vi "Pre-Build Action.vi"(6 "Top Level/Always Included VIs":path[](array[path]), 7 "Main Destination Path":path, 9 "Target Name":string, 10 "Build Specification Name":string, 11 "Project Path":path) -> (0 "error out":errorcluster)   [LabVIEW 2023]
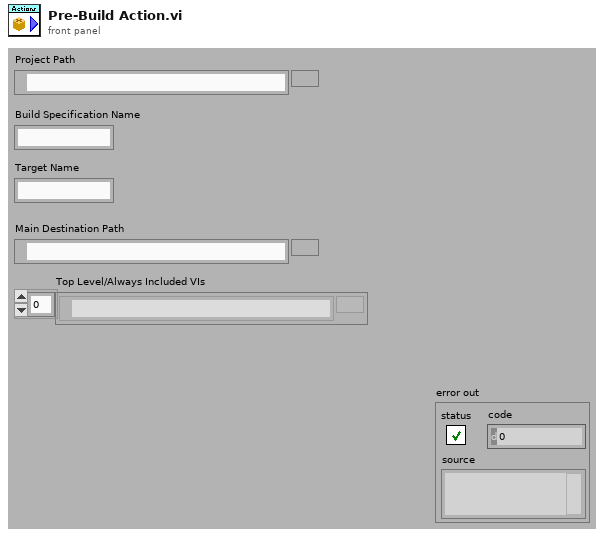
[diagram p1: front panel]
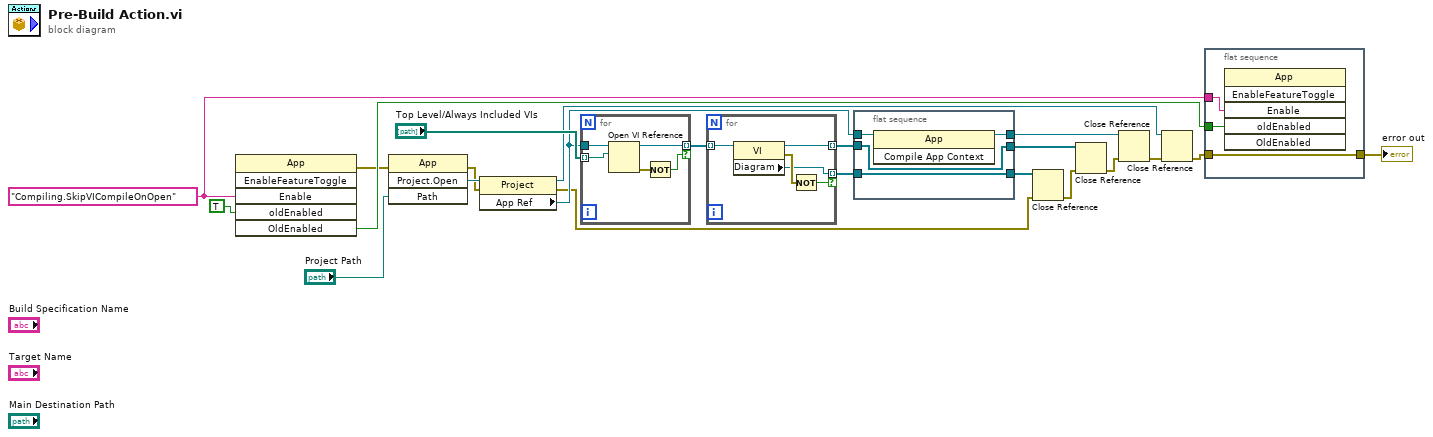
[diagram p0: block diagram]
diagram:
  w18 = "Compiling.SkipVICompileOnOpen" ("TokenName")
  n1 = invoke class="App" method="EnableFeatureToggle"("Enable"=w18, "oldEnabled"=TRUE ("Enable")) -> (error out=w16:errorcluster, "OldEnabled"=w17:bool)  [unwired: 4 in, 4 out]
  n2 = invoke class="App" method="Project.Open"(error in=w16, "Path"="Project Path") -> (error out=w20:errorcluster, "Project:Open"=w21:refnum<vi>)  [unwired: 2 in, 2 out]
  n3 = property class="Project"(reference=w21, error in=w20) -> (reference out=w5:refnum<vi>, error out=w4:errorcluster, "App Ref"=w11:refnum<vi>)
  n4 = for {
    tunnel: "Top Level/Always Included VIs" -> [w27] mode=indexing
    tunnel: [w26] -> w14 mode=indexing if=w24
    tunnel: w11 -> [w23]
    n5 = Open VI Reference(application reference (local)=w23, vi path=w27) -> (vi reference=w26:refnum<vi>, error out=w25:errorcluster)  [unwired: 4 in]
    n6 = Not(x=w25) -> (.not. x?=w24:bool)
  }
  n7 = for {
    tunnel: w14 -> [w32] mode=indexing
    tunnel: [w30] -> w12 mode=indexing if=w28
    tunnel: [w29] -> w13 mode=indexing
    n8 = property class="VI"(reference=w32) -> (reference out=w29:refnum<vi>, error out=w31:errorcluster, "Diagram"=w30:refnum<vi>)  [unwired: 1 in]
    n9 = Not(x=w31) -> (.not. x?=w28:bool)
  }
  n10 = flat-sequence {
    tunnel: [w36] -> w8
    tunnel: w13 -> [w36]
    tunnel: [w35] -> w10
    tunnel: w12 -> [w35]
    tunnel: w11 -> [w34]
    tunnel: [w33] -> w1
    frame #0 {
      n11 = invoke class="App" method="Compile App Context"(reference=w34) -> (reference out=w33:refnum<vi>)  [unwired: 2 in, 2 out]
    }
  }
  n12 = Close Reference(reference=w10, error in (no error)=w4) -> (error out=w9:errorcluster)
  n13 = Close Reference(reference=w8, error in (no error)=w9) -> (error out=w3:errorcluster)
  n14 = Close Reference(reference=w1, error in (no error)=w3) -> (error out=w2:errorcluster)
  n15 = Close Reference(reference=w5, error in (no error)=w2) -> (error out=w6:errorcluster)
  n16 = flat-sequence {
    tunnel: w18 -> [w39]
    tunnel: w17 -> [w38]
    tunnel: w6 -> [w37]
    tunnel: [w37] -> w7
    frame #0 {
      n17 = invoke class="App" method="EnableFeatureToggle"("Enable"=w39, "oldEnabled"=w38) -> ()  [unwired: 4 in, 6 out]
    }
  }
  "error out" <- w7
